vi "TEMPLATE.vi"() -> (2 "Msg Strategy":refnum<class "Msg Strategy.lvclass">)   [LabVIEW 2021, in "_Template.lvlib" / "Templates.lvlib" / "TEMPLATE Msg Strategy.lvlib"]
uses:
  TEMPLATE Msg Strategy.lvlib
  jettl/jettl/Msg Strategy/Msg Strategy.lvclass
  TEMPLATE Msg Strategy/TEMPLATE Msg Strategy.lvclass
  C:/git/jettl/jettl/jettl/Msg Strategy/Msg Strategy.lvclass
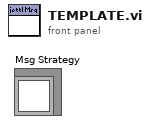
[diagram p1: front panel]
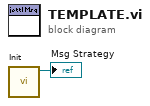
[diagram p0: block diagram]
diagram:
  n1 = call "Init.vi"() -> ("TEMPLATE Msg Strategy out"=→"Msg Strategy":refnum<class "TEMPLATE Msg Strategy.lvclass">)  [unwired: 11 in]
